vi "security.vi"() -> ()   [LabVIEW 2011]
uses:
  <vilib>/Utility/inputDevices.llb/closeKeyboard.vi
  <vilib>/Utility/inputDevices.llb/keyboardAcquire.vi
panel:
  out "Mode Panel":enum32{"Normal", "Add User", "Delete User"}(tab)
  out "String":string
  out "Postion of Sort":i32
  in  "Name":string
  in  "Passcode":string
  in  "Add User":bool
  in  "Delete":bool
  in  "User Index":dbl
  out "Users":cluster{"Name":string, "Passcode":string}[](array[cluster])
  in  "Mode":u16(ring) items=["Normal", "Add User", "Delete User"]
  in  "stop":bool
  # "Key the User's Index Number into the \nbox below and press OK.  You will be \nprompted to acknowledge user deletion"
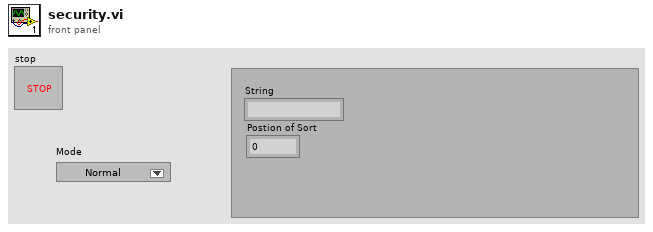
[diagram p1: front panel]
types:
  T1 = enum16{"open", "replace", "create", "open or create", "replace or create", "replace or create with confirmation"}
  T2 = enum16{"0", "1", "2", "3", "4", "5", "6", "7", "8", "9", "A", "B", "C", "D", "E", "F", "G", "H", "I", "J", "K", "L", "M", "N", "O", "P", "Q", "R", "S", "T", "U", "V", "W", "X", "Y", "Z", "F1", "F2", "F3", "F4", "F5", "F6", "F7", "F8", "F9", "F10", "F11", "F12", "F13", "F14", "F15", "ADD", "BACK", "BACKSLASH", "CAPITAL", "COMMA", "DECIMAL", "DELETE", "DIVIDE", "DOWN", "END", "EQUALS", "ESCAPE", "GRAVE (`)", "HOME", "INSERT", "LBRACKET", "LCONTROL", "LEFT", "L ALT", "LSHIFT", "LWIN", "MINUS", "MULTIPLY", "NEXT", "NUMLOCK", "NUMPAD_0", "NUMPAD_1", "NUMPAD_2", "NUMPAD_3", "NUMPAD_4", "NUMPAD_5", "NUMPAD_6", "NUMPAD_7", "NUMPAD_8", "NUMPAD_9", "PAUSE", "PERIOD", "PRIOR (PG UP)", "RBRACKET", "RCONTROL", "RETURN", "RIGHT", "R ALT", "RSHIFT", "RWIN", "SCROLL", "SEMICOLON", "SLASH", "SPACE", "SUBTRACT", "TAB", "UP", "ENTER (num pad)", "' (quote)"}[]
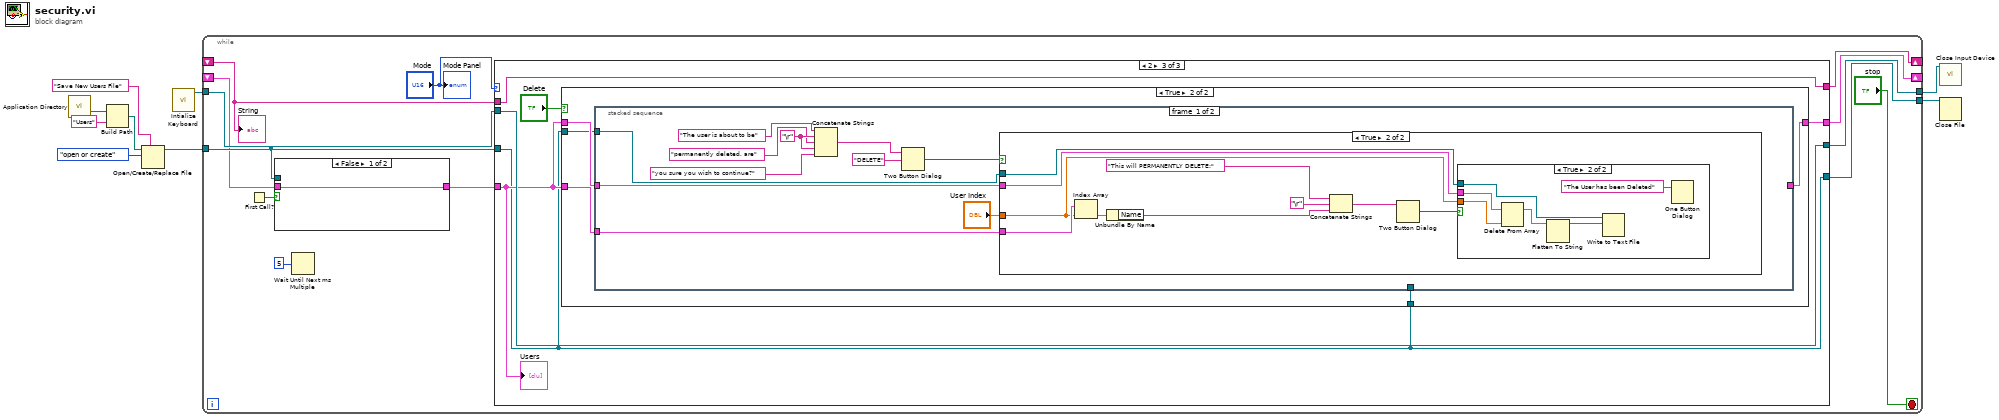
[diagram p0: block diagram]
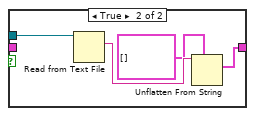
[diagram p2: hidden frame]
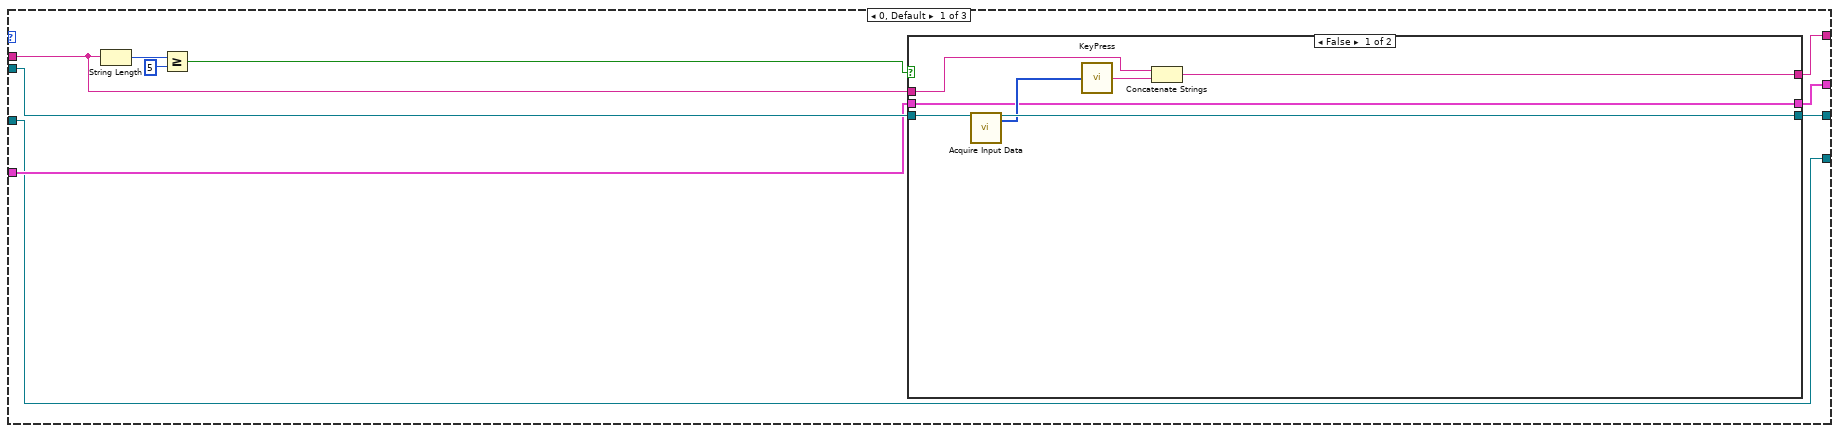
[diagram p3: hidden frame]
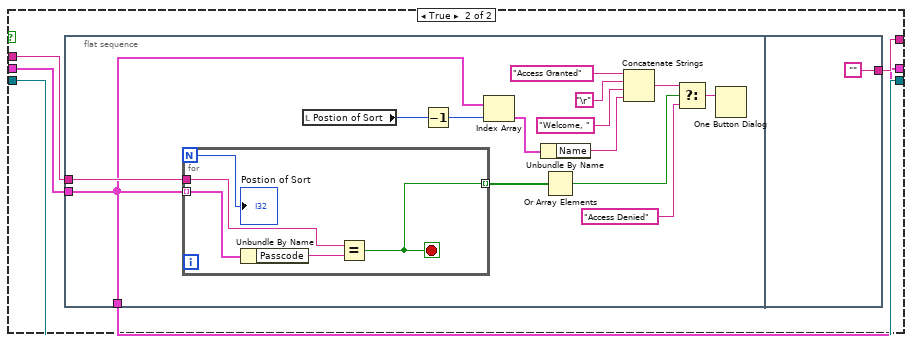
[diagram p4: hidden frame]
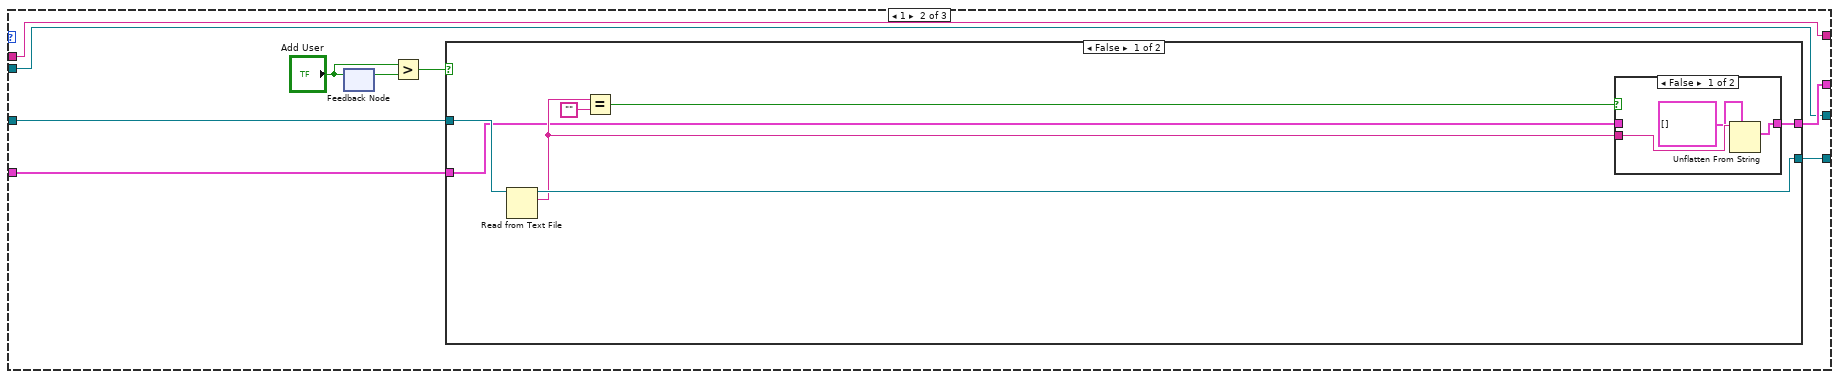
[diagram p5: hidden frame]
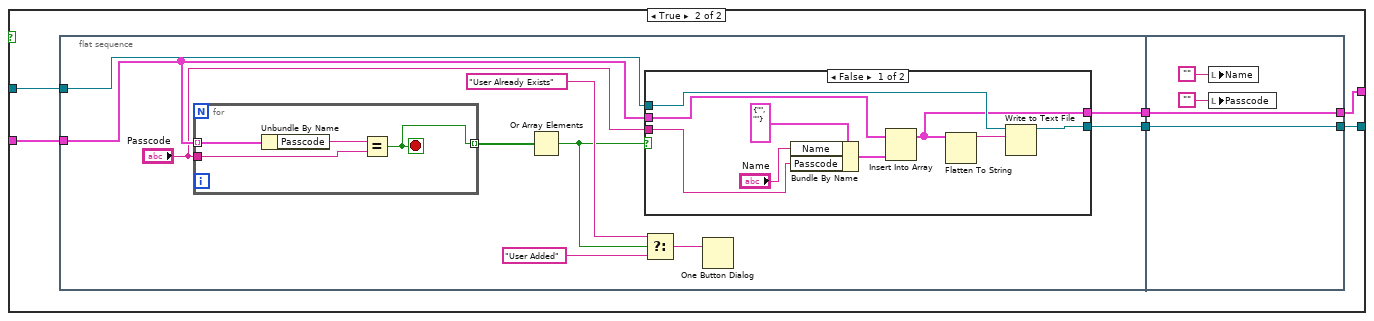
[diagram p7: hidden frame]
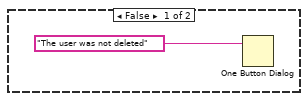
[diagram p10: hidden frame]
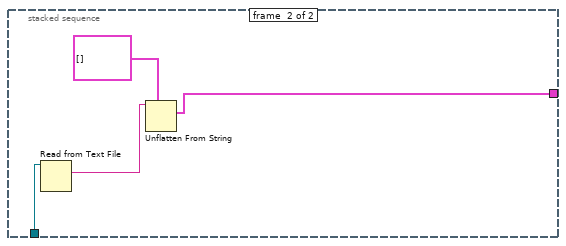
[diagram p12: hidden frame]
diagram:
  n1 = call <vilib>:"Application Directory.vi"() -> ("Application Directory"=w7:path)
  n2 = Build Path(base path=w7, name or relative path="Users") -> (appended path=w5:path)
  n3 = Open/Create/Replace File(file path (use dialog)=w5, prompt="Save New Users File", operation (0:open)=T1."open or create") -> (refnum out=w2:refnum<file>)  [unwired: 3 in, 2 out]
  n4 = call <vilib>:"Intialize Keyboard.vi"() -> ("device ID"=w9:refnum<k1>)  [unwired: 10 in, 1 out]
  n5 = while {
    tunnel: w9 -> [w22]
    tunnel: [w20] -> w8
    shift-right: [w19] -> _
    shift-left: _ -> [w17]
    tunnel: w2 -> [w12]
    tunnel: [w16] -> w1
    shift-right: [w15] -> _
    shift-left: _ -> [w10]
    stop <- "stop" stop-if-true
    n6 = First Call?() -> (First Call?: T/F=w13:bool)
    n7 = case shown="False" w13 {
      tunnel: w12 -> [_ w27]
      tunnel: [w23 w25] -> w11
      tunnel: w10 -> [w23 _]
      frame False {
      }
      frame True {
        n8 = Read from Text File(file (use dialog)=w27) -> (text=w26:string)  [unwired: 3 in, 3 out]
        n9 = Unflatten From String(type=cluster{"Name":string, "Passcode":string}[] [], binary string=w26) -> (value=w25:cluster{"Name":string, "Passcode":string}[])  [unwired: 3 in, 2 out]
      }
    }
    n10 = Wait Until Next ms Multiple(millisecond multiple=u32 5) -> ()  [unwired: 1 out]
    n11 = case shown="2" "Mode" {
      tunnel: w22 -> [w37 w71 w130]
      tunnel: [w36 w71 w130] -> w20
      tunnel: [w35 w70 w129] -> w19
      tunnel: w17 -> [w31 w70 w129]
      tunnel: w11 -> [w30 w72 w126]
      tunnel: w12 -> [w29 w75 w125]
      tunnel: [w29 w74 w125] -> w16
      tunnel: [w28 w73 w127] -> w15
      frame 0, Default {
        n12 = String Length(string=w31) -> (length=w34:i32)
        n13 = Greater Or Equal?(x=w34, y=5) -> (x >= y?=w32:bool)
        n14 = case shown="False" w32 {
          tunnel: w37 -> [w44 w49]
          tunnel: [w43 w49] -> w36
          tunnel: w31 -> [w42 w48]
          tunnel: [w41 w47] -> w35
          tunnel: w30 -> [w38 w46]
          tunnel: [w38 w45] -> w28
          frame False {
            n15 = call-poly <vilib>:"Acquire Input Data.vi"("device ID"=w44) -> ("device ID"=w43:refnum<k1>, "keys pressed"=w40:T2)  [unwired: 16 in, 1 out]
            n16 = call "KeyPress.vi"("keys pressed"=w40) -> ("Keys Found"=w39:string)
            n17 = Concatenate Strings(w42, w39) -> (w41:string)
          }
          frame True {
            n18 = flat-sequence {
              tunnel: w48 -> [w61]
              tunnel: w46 -> [w58]
              tunnel: [w58] -> w45
              tunnel: [""] -> w47
              frame #0 {
                n19 = for {
                  N -> [w64]
                  tunnel: w58 -> [w68] mode=indexing
                  tunnel: w61 -> [w66]
                  tunnel: [w65] -> w60 mode=indexing
                  stop <- w65 stop-if-true
                  n20 = Unbundle By Name(w68) -> ("Passcode"=w67:string)
                  n21 = Equal?(x=w66, y=w67) -> (x = y?=w65:bool)
                  "Postion of Sort" <- w64
                }
                n22 = local read "Postion of Sort"() -> (w51:i32)
                n23 = Decrement(x=w51) -> (x-1=w50:i32)
                n24 = Index Array(array=w58, index=w50) -> (element=w57:cluster{"Name":string, "Passcode":string})
                n25 = Unbundle By Name(w57) -> ("Name"=w55:string)
                n26 = Or Array Elements(Boolean array=w60) -> (logical OR=w59:bool)
                n27 = Concatenate Strings("Access Granted" ("message"), "\r", "Welcome, " ("string"), w55) -> (w52:string)
                n28 = Select(t=w52, s=w59, f="Access Denied" ("message")) -> (s? t:f=w62:string)
                n29 = One Button Dialog(message=w62) -> ()  [unwired: 1 in, 1 out]
              }
              frame #1 {
              }
            }
          }
        }
      }
      frame 1 {
        n30 = feedback #1() -> (w77:bool)  [unwired: 1 in]
        n31 = feedback-in #1("Add User") -> ()
        n32 = Greater?(x="Add User", y=w77) -> (0:w76:bool)
        n33 = case shown="False" w76 {
          tunnel: w72 -> [w79 w92]
          tunnel: [w83 w93] -> w73
          tunnel: w75 -> [w85 w95]
          tunnel: [w84 w94] -> w74
          frame False {
            n34 = Read from Text File(file (use dialog)=w85) -> (refnum out=w84:refnum<file>, text=w81:string)  [unwired: 3 in, 2 out]
            n35 = Equal?(x=w81, y="") -> (x = y?=w82:bool)
            n36 = case shown="False" w82 {
              tunnel: w81 -> [w88 _]
              tunnel: [w86 w89] -> w83
              tunnel: w79 -> [_ w89]
              frame False {
                n37 = Unflatten From String(type=cluster{"Name":string, "Passcode":string}[] [], binary string=w88) -> (value=w86:cluster{"Name":string, "Passcode":string}[])  [unwired: 3 in, 2 out]
              }
              frame True {
              }
            }
          }
          frame True {
            n38 = flat-sequence {
              tunnel: w95 -> [w105]
              tunnel: w92 -> [w102]
              tunnel: [w104] -> w91
              tunnel: [w103] -> w90
              tunnel: [w123] -> w93
              tunnel: [w124] -> w94
              tunnel: w91 -> [w124]
              tunnel: w90 -> [w123]
              frame #0 {
                n39 = for {
                  tunnel: w102 -> [w120] mode=indexing
                  tunnel: "Passcode" -> [w119]
                  tunnel: [w117] -> w101 mode=indexing
                  stop <- w117 stop-if-true
                  n40 = Unbundle By Name(w120) -> ("Passcode"=w118:string)
                  n41 = Equal?(x=w118, y=w119) -> (x = y?=w117:bool)
                }
                n42 = Or Array Elements(Boolean array=w101) -> (logical OR=w96:bool)
                n43 = case shown="False" w96 {
                  tunnel: w105 -> [w111 w116]
                  tunnel: [w110 w116] -> w104
                  tunnel: [w108 w115] -> w103
                  tunnel: w102 -> [w107 w115]
                  tunnel: "Passcode" -> [w106 _]
                  frame False {
                    n44 = Bundle By Name(cluster=cluster{"Name":string, "Passcode":string} {"Name"="", "Passcode"=""} ("User Data"), "Name"="Name", "Passcode"=w106) -> (w114:cluster{"Name":string, "Passcode":string})
                    n45 = Insert Into Array(array=w107, new element=w114) -> (w108:cluster{"Name":string, "Passcode":string}[])  [unwired: 1 in]
                    n46 = Flatten To String(anything=w108) -> (data string=w109:string)  [unwired: 3 in, 2 out]
                    n47 = Write to Text File(file (use dialog)=w111, text=w109) -> (refnum out=w110:refnum<file>)  [unwired: 2 in, 2 out]
                  }
                  frame True {
                    # "User Alreadu Exists; do nothing"
                  }
                }
                n48 = Select(t="User Already Exists" ("message"), s=w96, f="User Added") -> (s? t:f=w98:string)
                n49 = One Button Dialog(message=w98) -> ()  [unwired: 1 in, 1 out]
              }
              frame #1 {
                n50 = local write "Name"("") -> ()
                n51 = local write "Passcode"("") -> ()
              }
            }
          }
        }
      }
      frame 2 {
        n52 = case shown="True" "Delete" {
          tunnel: w126 -> [w131 w136]
          tunnel: [w131 w135] -> w127
          tunnel: w126 -> [_ w134]
          tunnel: w125 -> [_ w133]
          tunnel: w125 -> [_ w132]
          frame False {
          }
          frame True {
            n53 = stacked-sequence {
              tunnel: w136 -> [w140 _]
              tunnel: [_ w165] -> w135
              tunnel: w134 -> [w138 _]
              tunnel: w133 -> [w137 _]
              tunnel: w132 -> [_ w168]
              frame #0 {
                w146 = "\r"
                n54 = Concatenate Strings("The user is about to be" ("message"), w146, "permanently deleted, are" ("message"), w146, "you sure you wish to continue?" ("message")) -> (w143:string)
                n55 = Two Button Dialog(message=w143, 2:"DELETE" ("T button name (\"OK\")")) -> (T button?=w141:bool)  [unwired: 1 in]
                n56 = case shown="True" w141 {
                  tunnel: w140 -> [_ w158]
                  tunnel: "User Index" -> [_ w153]
                  tunnel: w138 -> [_ w154]
                  tunnel: w137 -> [_ w149]
                  frame False {
                    n57 = One Button Dialog(message="The user was not deleted") -> ()  [unwired: 1 in, 1 out]
                  }
                  frame True {
                    n58 = Index Array(array=w154, index=w153) -> (element=w152:cluster{"Name":string, "Passcode":string})
                    n59 = Unbundle By Name(w152) -> ("Name"=w151:string)
                    n60 = Concatenate Strings("This will PERMANENTLY DELETE:" ("string"), "\r", w151) -> (w150:string)
                    n61 = Two Button Dialog(message=w150) -> (T button?=w157:bool)  [unwired: 2 in]
                    n62 = case shown="True" w157 {
                      tunnel: w158 -> [_ w164]
                      tunnel: w153 -> [_ w163]
                      tunnel: w149 -> [_ w159]
                      frame False {
                      }
                      frame True {
                        n63 = Delete From Array(array=w164, index=w163) -> (array with subset deleted=w161:cluster{"Name":string, "Passcode":string}[])  [unwired: 1 in, 1 out]
                        n64 = Flatten To String(anything=w161) -> (data string=w160:string)  [unwired: 3 in, 2 out]
                        n65 = Write to Text File(file (use dialog)=w159, text=w160) -> ()  [unwired: 2 in, 3 out]
                        n66 = One Button Dialog(message="The User has been Deleted") -> ()  [unwired: 1 in, 1 out]
                      }
                    }
                  }
                }
              }
              frame #1 {
                n67 = Read from Text File(file (use dialog)=w168) -> (text=w167:string)  [unwired: 3 in, 3 out]
                n68 = Unflatten From String(type=cluster{"Name":string, "Passcode":string}[] [], binary string=w167) -> (value=w165:cluster{"Name":string, "Passcode":string}[])  [unwired: 3 in, 2 out]
              }
            }
          }
        }
        "Users" <- w126
      }
    }
    "String" <- w17
    "Mode Panel" <- "Mode"
  }
  n69 = call-poly <vilib>:"Close Input Device.vi"("device ID"=w8) -> ()  [unwired: 9 in, 1 out]
  n70 = Close File(refnum=w1) -> ()  [unwired: 1 in, 2 out]
